vi "GetTriggerTime.vi"(8 "error in (no error)":errorcluster, 11 "TriggerIndex (1)":u8=1) -> (0 "error out":errorcluster, 3 "TriggerTime [ns]":i64)   [LabVIEW 2014]
uses:
  <vilib>/httpClient/LabVIEWHTTPClient.lvlib
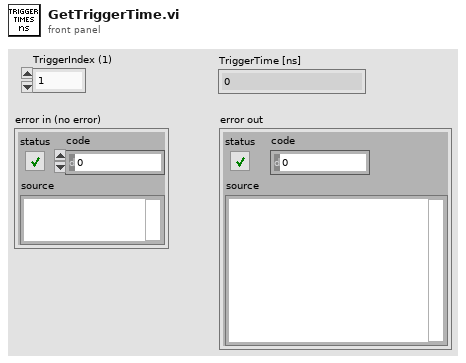
[diagram p1: front panel]
types:
  T1 = typedef "LabVIEWHTTPClient.lvlib/ClientHandle.ctl" = refnum<k1>
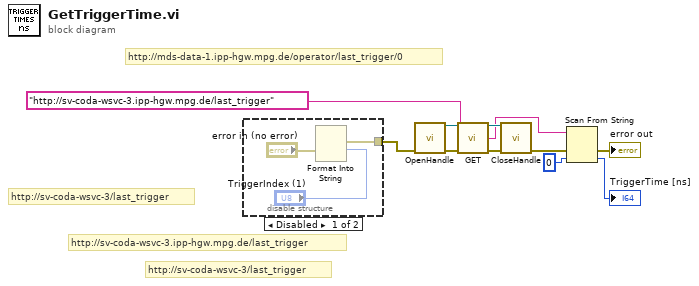
[diagram p0: block diagram]
diagram:
  # "http://sv-coda-wsvc-3/last_trigger"
  # "http://sv-coda-wsvc-3.ipp-hgw.mpg.de/last_trigger"
  # "http://sv-coda-wsvc-3/last_trigger"
  # "http://mds-data-1.ipp-hgw.mpg.de/operator/last_trigger/0"
  n1 = disable-structure shown="Disabled" {
    disable-tunnel: [w12 _] -> w3
    frame Disabled {
      n2 = Format Into String(error in="error in (no error)", "TriggerIndex (1)") -> (error out=w12:errorcluster)  [unwired: 3 in, 1 out]
    }
    frame Enabled {
    }
  }
  n3 = call <vilib>:"OpenHandle.vi"("error in (no error)"=w3) -> ("client handle out"=w8:T1, "error out"=w2:errorcluster)  [unwired: 13 in]
  n4 = call <vilib>:"GET.vi"("client handle"=w8, "url"="http://sv-coda-wsvc-3.ipp-hgw.mpg.de/last_trigger", "error in (no error)"=w2) -> ("client handle out"=w9:T1, "body"=w5:string, "error out"=w10:errorcluster)  [unwired: 9 in, 1 out]
  n5 = call <vilib>:"CloseHandle.vi"("client handle"=w9, "error in (no error)"=w10) -> ("error out"=w11:errorcluster)  [unwired: 13 in]
  n6 = Scan From String(input string=w5, error in=w11, default 1=i64 0 ("default (0 I32)")) -> (error out=→"error out":errorcluster, output 1=→"TriggerTime [ns]":i64)  [unwired: 2 in, 2 out]
